vi "Create Port.vi"(0 "Node name":string, 5 "size":i16 caption="x", 7 "x":i16, 9 "y":i16) -> (4 "FSM.Port":refnum<class "FSM.Port.lvclass">)   [LabVIEW 2020, in "FSM.Port.lvclass"]
uses:
  FSM.Port.lvclass
  FSM.Port.lvclass/FSM.Port.ctl
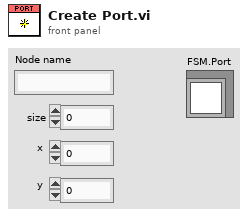
[diagram p1: front panel]
types:
  T1 = cluster{"left":i16, "top":i16, "right":i16, "bottom":i16}
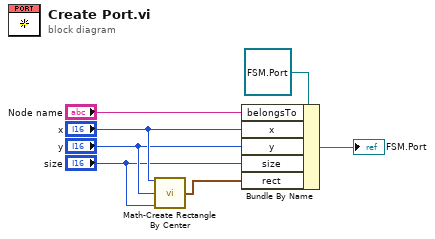
[diagram p0: block diagram]
diagram:
  n1 = call "Math-Create Rectangle By Center.vi"("x"="x", "y"="y", "size"="size") -> ("rect"=w1:T1)  [unwired: 12 in]
  n2 = Bundle By Name(cluster=refnum<class "FSM.Port.lvclass"> refnum ("FSM.Port"), "belongsTo"="Node name", "x"="x", "y"="y", "size"="size", "rect"=w1) -> (→"FSM.Port":refnum<class "FSM.Port.lvclass">)
